vi "To And From String Array Test.vi"() -> ()   [LabVIEW 2015, in "Counter Tests.lvlib"]
uses:
  Counter Tests.lvlib
  Config/Counter Config.lvclass
  <vilib>/NI/Tag Bus/tag/Data Type.ctl
  <vilib>/NI/Tag Bus Module Framework/channel/channel classification.ctl
  <vilib>/NI/Tag Bus/tag/tag descriptor.lvclass
  <vilib>/NI/Tag Bus Module Framework/channel/TBM channel.lvclass
panel:
  out "error out":errorcluster
  out "Pass":bool
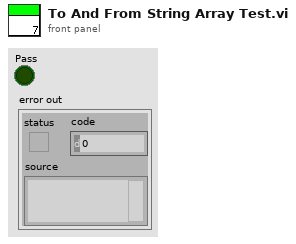
[diagram p1: front panel]
types:
  T1 = typedef "TBM channel.lvclass/channel classification.ctl" = enum16{"input data", "output data", "processing parameter", "processing result"}
  T2 = typedef "tag bus.lvlib/tag descriptor.lvclass/Data Type.ctl" = enum16{"Double", "Single", "I64", "I32", "I16", "I8", "U64", "U32", "U16", "U8", "Boolean", "String", "Array of Double", "Array of Single", "Array of I64", "Array of I32", "Array of I16", "Array of I8", "Array of U64", "Array of U32", "Array of U16", "Array of U8", "Array of Boolean", "Array of String"}
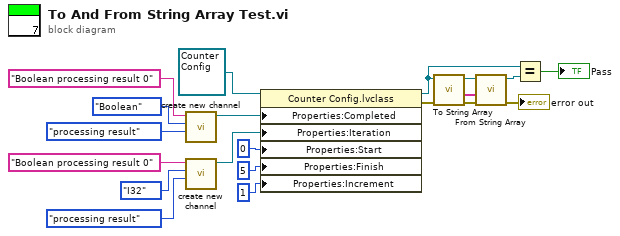
[diagram p0: block diagram]
diagram:
  n1 = call <vilib>:"create new channel.vi"("channel classification"=channel_classification."processing result", "data type"=Data_Type."Boolean" ("Data Type"), "channel name"="Boolean processing result 0" ("Completed Tag name")) -> ("channel"=w4:refnum<class "TBM channel.lvclass">)  [unwired: 8 in]
  n2 = call <vilib>:"create new channel.vi"("channel classification"=channel_classification."processing result", "data type"=Data_Type."I32" ("Data Type"), "channel name"="Boolean processing result 0" ("Iteration Tag Name")) -> ("channel"=w7:refnum<class "TBM channel.lvclass">)  [unwired: 8 in]
  n3 = property class="Counter Config.lvclass"(reference=refnum<class "Counter Config.lvclass"> refnum ("Counter Config.lvclass"), "Properties:Completed"=w4, "Properties:Iteration"=w7, "Properties:Start"=0 ("Start"), "Properties:Finish"=5 ("Finish"), "Properties:Increment"=1 ("Increment")) -> (reference out=w2:refnum<class "Counter Config.lvclass">, error out=w1:errorcluster)  [unwired: 1 in]
  n4 = call-dynamic "To String Array.vi"("error in (no error)"=w1, "Counter Config in"=w2) -> ("error out"=w18:errorcluster, "Step String Array"=w19:string[], "Counter Config out"=w20:refnum<class "Counter Config.lvclass">)  [unwired: 7 in]
  n5 = call-dynamic "From String Array.vi"("error in (no error)"=w18, "String Array"=w19, "Counter Config in"=w20) -> ("error out"=→"error out":errorcluster, "Counter Config out"=w17:refnum<class "Counter Config.lvclass">)  [unwired: 7 in]
  n6 = Equal?(x=w2, y=w17) -> (x = y?=→"Pass":bool)
